vi "控制方式转换.vi"() -> ()   [LabVIEW 2010]
panel:
  in  "停  止":bool
  in  "控制方式选择":bool
  in  "电机转速":dbl(slide) scale=0.0..1000.0
  # "手动   自动"
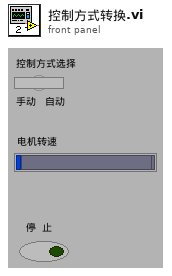
[diagram p1: front panel]
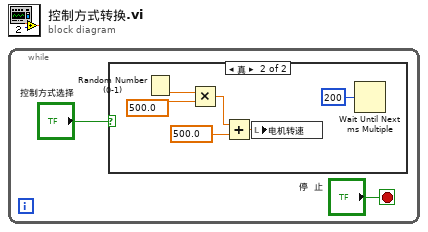
[diagram p0: block diagram]
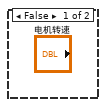
[diagram p2: hidden frame]
diagram:
  n1 = while {
    stop <- "停  止" stop-if-true
    n2 = case shown="真" "控制方式选择" {
      frame False {
      }
      frame True {
        n3 = Random Number (0-1)() -> (number: 0 to 1=w8:dbl)
        n4 = Multiply(x=w8, y=500.0) -> (x*y=w6:dbl)
        n5 = Add(x=w6, y=500.0) -> (x+y=w4:dbl)
        n6 = local write "电机转速"(w4) -> ()
        n7 = Wait Until Next ms Multiple(millisecond multiple=u32 200) -> ()  [unwired: 1 out]
      }
    }
  }
